vi "CCInitializeDICOMAttributes.vi"(8 "error in (no error)":errorcluster, 11 "filename":string) -> (0 "error out":errorcluster)   [LabVIEW 2013, in "ClearCanvasLibrary.lvlib"]
uses:
  Controls/Enum Variables.ctl
  C:/Users/Simon/SkyDrive/LabView/2013/DM2020/DICOM/ClearCanvasNewBuild/ClearCanvas.Dicom.dll
  ClearCanvasNewBuild/ClearCanvas.Dicom.dll
  ClearCanvasLibrary.lvlib
  main.lvlib
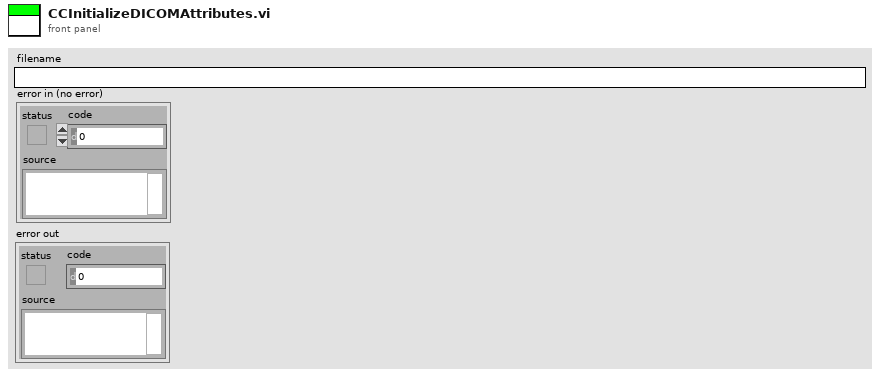
[diagram p1: front panel]
types:
  T1 = typedef "main.lvlib/Enum Variables.ctl" = enum16{"SetAcqFilter", "GetAcqFilter", "Set Filter", "Get Filter", "Set Height", "Get Height", "Set Blue Pressure", "Get Blue Pressure", "Set Red Pressure", "Get Red Pressure", "Init", "Reset Pressure", "Set Red Cursors", "Get Red Cursors", "Set Blue Cursors", "Get Blue Cursors", "Set Language", "Get Language", "Set Active Graphs", "Get ActiveGraphs", "Set Method", "Get Method", "Set Encryption", "Get Encryption", "Set ExcelVersion", "Get ExcelVersion", "Set itemTags", "Get itemTags", "Set Attributes", "Get Attributes", "Set DICOM Avail", "Get DICOM Avail", "Set DICOM Encode", "Get DICOM Encode", "Set JournalExport", "Get JournalExport", "Set Sequence", "Get Sequence", "Set DAQ Connected", "Get DAQ Connected", "Set Current Graph", "Get Current Graph", "Set General Settings", "Get Hyphenation", "Set Arm Calc Method", "Get Arm Calc Method", "Set Dicom Tags", "Get Dicom Tags"}
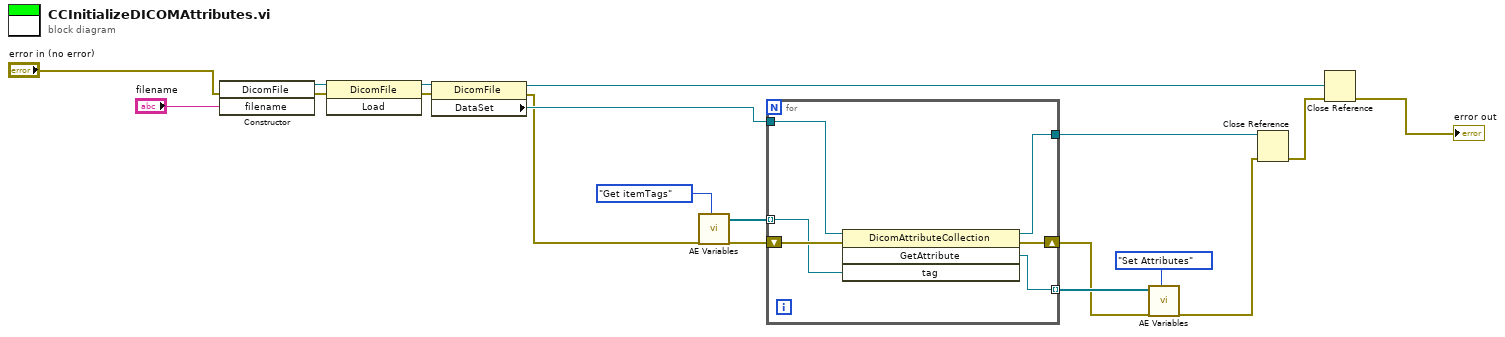
[diagram p0: block diagram]
diagram:
  n1 = constructor class="DicomFile"(error in="error in (no error)", "filename"="filename") -> (reference out=w19:refnum<k24>, error out=w16:errorcluster)  [unwired: 2 in, 2 out]
  n2 = invoke class="DicomFile" method="Load"(reference=w19, error in=w16) -> (reference out=w17:refnum<k24>, error out=w15:errorcluster)  [unwired: 1 in, 1 out]
  n3 = property class="DicomFile"(reference=w17, error in=w15) -> (reference out=w14:refnum<k24>, error out=w6:errorcluster, "DataSet"=w13:refnum<k24>)
  n4 = call "AE Variables.vi"("error in (no error)"=w6, "Action"=Enum_Variables."Get itemTags") -> ("itemTags .net"=w8:refnum<k24>[], "error out"=w7:errorcluster)  [unwired: 9 in, 7 out]
  n5 = for {
    tunnel: w13 -> [w22]
    tunnel: w8 -> [w21] mode=indexing
    tunnel: [w25] -> w11 mode=indexing
    shift-right: [w24] -> w4
    shift-left: w7 -> [w23]
    tunnel: [w20] -> w5
    n6 = invoke class="DicomAttributeCollection" method="GetAttribute"(reference=w22, error in=w23, "tag"=w21) -> (reference out=w20:refnum<k24>, error out=w24:errorcluster, "GetAttribute"=w25:refnum<k24>)  [unwired: 1 in, 1 out]
  }
  n7 = call "AE Variables.vi"("VariantIn"=w11, "error in (no error)"=w4, "Action"=Enum_Variables."Set Attributes") -> ("error out"=w1:errorcluster)  [unwired: 8 in, 8 out]
  n8 = Close Reference(reference=w5, error in (no error)=w1) -> (error out=w3:errorcluster)
  n9 = Close Reference(reference=w14, error in (no error)=w3) -> (error out=→"error out":errorcluster)
